vi "test_awgMemReplay_main.vi"() -> ()   [LabVIEW 2016]
uses:
  <vilib>/rvi/DesktopExecutionNode/DesktopExecutionNode.xnode
  <vilib>/rvi/DesktopExecutionNode/Execution/niFpgaDEN_Execute.vi
panel:
  out "XY Graph":cluster{i32[], dbl[]}(graph)
  out "debug":T1(array[cluster])
  in  "maxCount":u16
  out "Array":T2(array[cluster])
  in  "doStep":bool
  in  "clocks":T3
  in  "periodic":bool
  in  "reset":bool
  out "Progress":dbl(slide) scale=0.0..1.0
  in  "Simulation ticks":i32=10000
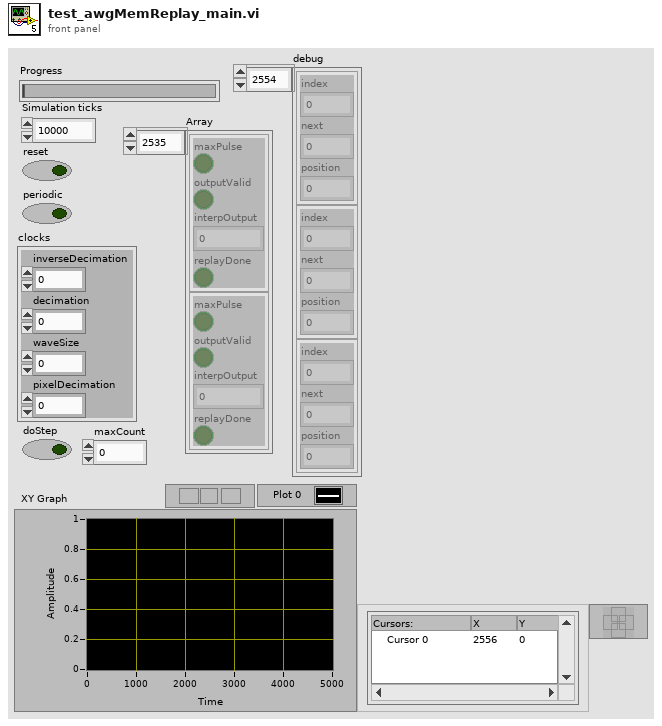
[diagram p1: front panel]
types:
  T1 = cluster{"index":u16, "next":u16, "position":fxp<+,22,0>}[]
  T2 = cluster{"maxPulse":bool, "outputValid":bool, "interpOutput":fxp<+/-,19,2>, "replayDone":bool}[]
  T3 = cluster{"inverseDecimation":fxp<+,22,0>, "decimation":u16, "waveSize":u16, "pixelDecimation":u16}
  T4 = cluster{"index":u16, "next":u16, "position":fxp<+,22,0>}
  T5 = cluster{"maxPulse":bool, "outputValid":bool, "interpOutput":fxp<+/-,19,2>, "replayDone":bool}
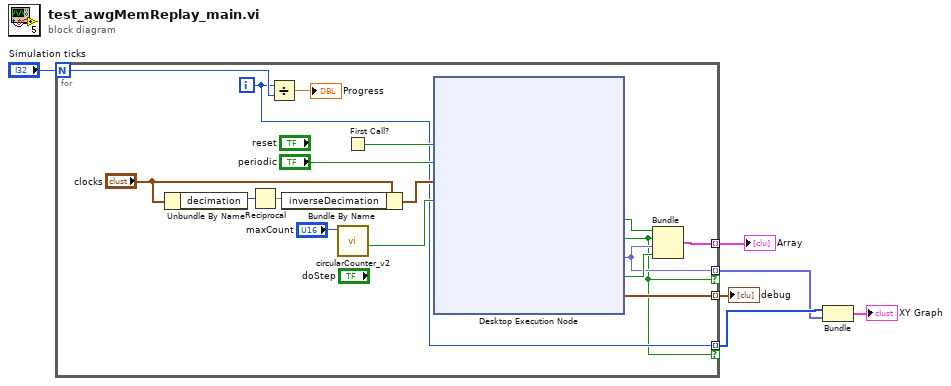
[diagram p0: block diagram]
diagram:
  n1 = for {
    N: "Simulation ticks" -> [w22]
    tunnel: [w18] -> w5 mode=indexing
    tunnel: [w10] -> w4 mode=indexing
    tunnel: [w9] -> w2 mode=indexing if=w7
    tunnel: [w8] -> w3 mode=indexing if=w7
    i -> [w8]
    n2 = Unbundle By Name("clocks") -> ("decimation"=w14:u16)
    n3 = Reciprocal(x=w14) -> (1/x=w15:dbl)
    n4 = Divide(x=w8, y=w22) -> (x/y=→"Progress":dbl)
    n5 = Bundle By Name(cluster="clocks", "inverseDecimation"=w15) -> (w12:T3)
    n6 = call "circularCounter_v2.vi"("maxCount"="maxCount") -> ("maxPulse"=w16:bool)  [unwired: 7 in, 3 out]
    n7 = First Call?() -> (First Call?: T/F=w11:bool)
    n8 = xnode "Desktop Execution Node"("reset"=w11, "periodic"="periodic", "clocks"=w12, "doStep"=w16) -> ("maxPulse"=w20:bool, "outputValid"=w7:bool, "interpOutput"=w9:fxp<+/-,19,2>, "replayDone"=w19:bool, "debug"=w10:T4)  [unwired: 1 in, 1 out]
    n9 = Bundle("maxPulse"=w20, "outputValid"=w7, "interpOutput"=w9, "replayDone"=w19) -> (w18:T5)  [unwired: 1 in]
  }
  "Array" <- w5
  "debug" <- w4
  n10 = Bundle(w3, w2) -> (→"XY Graph":cluster{i32[], fxp<+/-,19,2>[]})  [unwired: 1 in]
